vi "Check Error.vi"(8 "error in":errorcluster, 10 "timeout":u32=200, 11 "VISA resource name in":refnum<visa-resource-name>) -> (0 "error out":errorcluster, 1 "Message":string, 2 "status code":u8, 3 "VISA resource name out":refnum<visa-resource-name>, 4 "Status":T1)   [LabVIEW 2023, in "Digikrom DK24x.lvlib"]
doc: "Reads and decodes the instrument status bytes that follow every command. If there is an error condition, this VI will signal it."
uses:
  Digikrom DK24x.lvlib
panel:
  out "cancel byte":u8
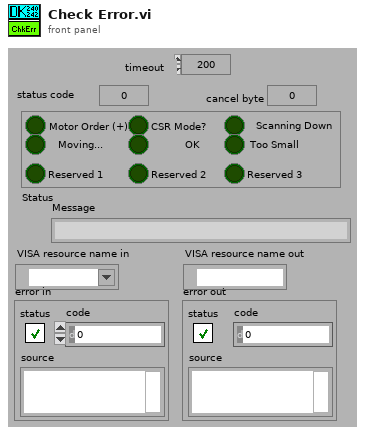
[diagram p1: front panel]
types:
  T1 = cluster{"Motor Order?":bool, "Reserved 1":bool, "CSR Mode?":bool, "Reserved 2":bool, "Scanning Up?":bool, "Too Large?":bool, "Already There?":bool, "Invalid Value?":bool, "Reserved 3":bool}
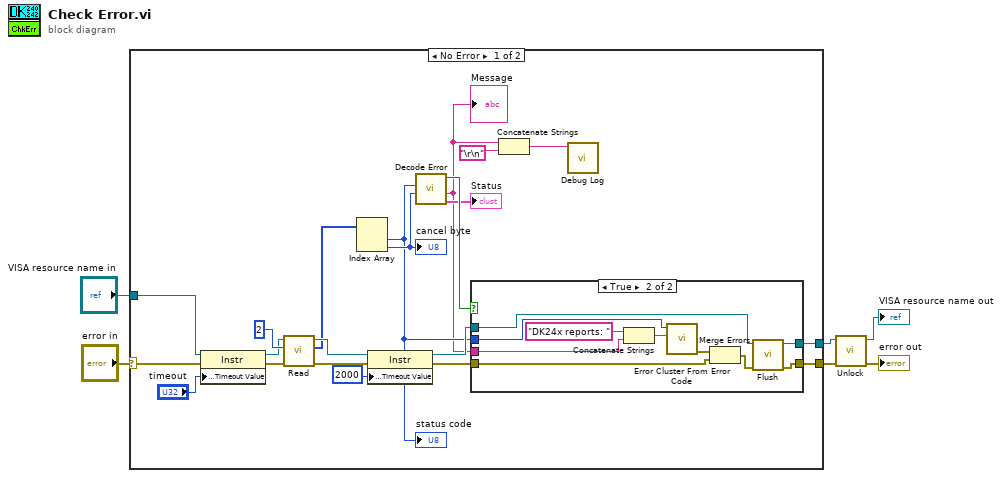
[diagram p0: block diagram]
diagram:
  n1 = case shown="No Error" "error in" {
    selector: "error in" -> [w10 w41]
    tunnel: [w27 w40] -> w2
    tunnel: "VISA resource name in" -> [w22 w40]
    tunnel: [w11 w41] -> w4
    frame No Error {
      n2 = property class="Instr"(reference=w22, error in=w10, "General Settings:Timeout Value"="timeout") -> (reference out=w21:refnum<visa-resource-name>, error out=w26:errorcluster)
      n3 = call "Read.vi"("error in (no error)"=w26, "response size"=u8 2, "VISA resource name"=w21) -> ("error out"=w25:errorcluster, "response array"=w16:u8[], "VISA resource name out"=w20:refnum<visa-resource-name>)  [unwired: 6 out]
      n4 = Index Array(array=w16) -> (element #1=w14:u8, element #2=w15:u8)  [unwired: 2 in]
      "status code" <- w14
      "cancel byte" <- w15
      n5 = property class="Instr"(reference=w20, error in=w25, "General Settings:Timeout Value"=u32 2000) -> (reference out=w18:refnum<visa-resource-name>, error out=w19:errorcluster)
      n6 = call "Decode Error.vi"("cancel byte"=w15, "status byte"=w14) -> ("Status"=→"Status":T1, "Error message"=w9:string, "Error occured?"=w13:bool)  [unwired: 7 out]
      "Message" <- w9
      n7 = case shown="True" w13 {
        tunnel: [w28 w37] -> w11
        tunnel: w19 -> [w28 w35]
        tunnel: w18 -> [w29 w38]
        tunnel: [w29 w39] -> w27
        tunnel: w14 -> [_ w32]
        tunnel: w9 -> [_ w33]
        frame False {
        }
        frame True {
          n8 = Concatenate Strings("DK24x reports: ", w33) -> (w31:string)
          n9 = call <vilib>:"Error Cluster From Error Code.vi"("error message (\"\")"=w31, "error code (0)"=w32) -> ("error out"=w30:errorcluster)  [unwired: 2 in, 5 out]
          n10 = Merge Errors(w30, w35) -> (w36:errorcluster)
          n11 = call "Flush.vi"("error in (no error)"=w36, "VISA resource name"=w38) -> ("error out"=w37:errorcluster, "VISA resource name out"=w39:refnum<visa-resource-name>)  [unwired: 8 out]
        }
      }
      n12 = Concatenate Strings(w9, "\r\n") -> (w8:string)
      n13 = call "Debug Log.vi"("Message"=w8) -> ()  [unwired: 2 in, 9 out]
    }
    frame Error {
    }
  }
  n14 = call "Unlock.vi"("error in"=w4, "VISA resource name"=w2) -> ("error out"=→"error out":errorcluster, "VISA resource name out"=→"VISA resource name out":refnum<visa-resource-name>)  [unwired: 8 out]
